vi "Edit Row (Variant).vi"(6 "Row Index":i32, 7 "image path":path, 8 "error in (no error)":errorcluster, 9 "New Row Data (or multi rows)":variant[][](array[variant]), 11 "DataGrid.lvlib:DataTable.lvclass 2":refnum<class "DataTable.lvclass">) -> (0 "error out":errorcluster, 3 "DataGrid.lvlib:DataTable.lvclass 2":refnum<class "DataTable.lvclass">)   [LabVIEW 2013, in "DataGrid.lvlib" / "DataTable.lvclass"]
doc: "Edits a row by simply replacing it with another row (or series of row) to essentially replace and insert at that location in the datatable."
uses:
  DataTable.lvclass
  DataTable.lvclass/DataTable.ctl
  System.Data
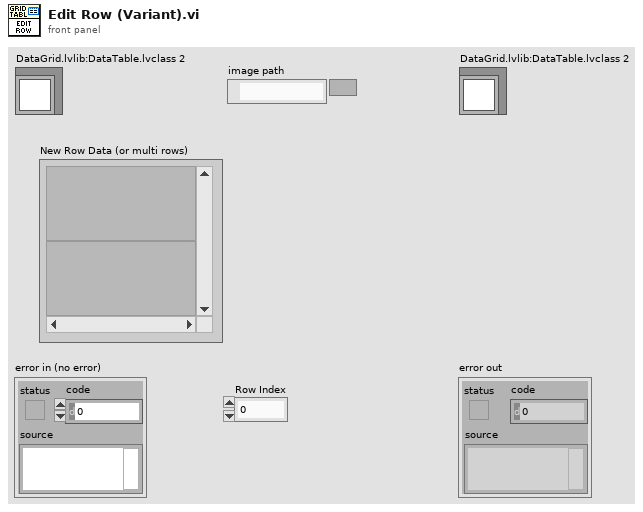
[diagram p1: front panel]
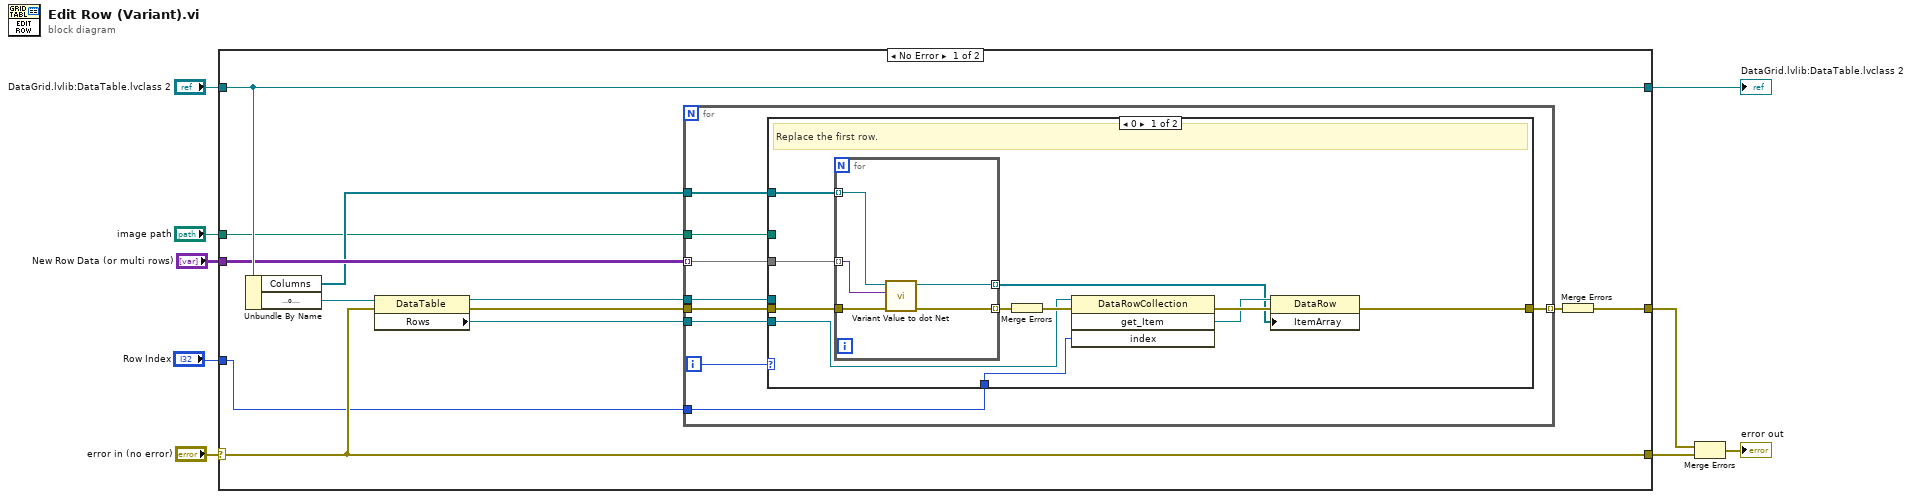
[diagram p0: block diagram]
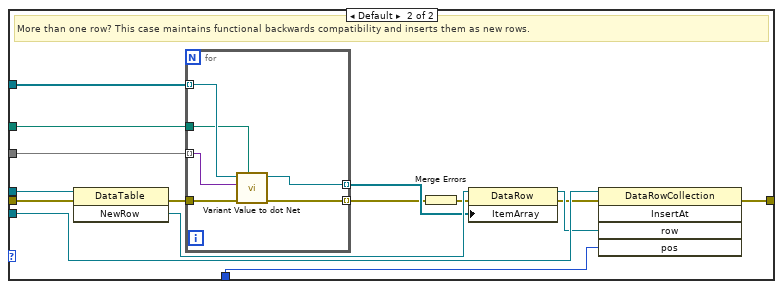
[diagram p2: hidden frame]
diagram:
  n1 = case shown="No Error" "error in (no error)" {
    selector: "error in (no error)" -> [w19 w69]
    tunnel: [w19 w69] -> w8
    tunnel: [w20 w68] -> w6
    tunnel: "DataGrid.lvlib:DataTable.lvclass 2" -> [w20 w68]
    tunnel: "New Row Data (or multi rows)" -> [w18 _]
    tunnel: [w16 _] -> w3
    tunnel: "Row Index" -> [w11 _]
    tunnel: "image path" -> [w10 _]
    frame No Error {
      n2 = Unbundle By Name(w20) -> ("Columns"=w15:refnum<class "GridColumn.lvclass">[], "DataTable"=w17:refnum<k24>)
      n3 = property class="DataTable"(reference=w17, error in=w19) -> (reference out=w14:refnum<k24>, error out=w13:errorcluster, "Rows"=w12:refnum<k24>)
      n4 = for {
        tunnel: w12 -> [w29]
        tunnel: w14 -> [w30]
        tunnel: [w28] -> w21 mode=indexing
        tunnel: w18 -> [w27] mode=indexing
        tunnel: w13 -> [w26]
        tunnel: w15 -> [w25]
        tunnel: w11 -> [w24]
        tunnel: w10 -> [w22]
        i -> [w23]
        n5 = case shown="0" w23 {
          tunnel: w30 -> [_ w61]
          tunnel: w29 -> [w36 w60]
          tunnel: [w31 w59] -> w28
          tunnel: w27 -> [w40 w58]
          tunnel: w26 -> [w39 w50]
          tunnel: w25 -> [w41 w49]
          tunnel: w24 -> [w35 w48]
          tunnel: w22 -> [_ w47]
          frame 0 {
            # "Replace the first row."
            n6 = for {
              tunnel: w40 -> [w46] mode=indexing
              tunnel: [w45] -> w32 mode=indexing
              tunnel: w39 -> [w44]
              tunnel: [w43] -> w38 mode=indexing
              tunnel: w41 -> [w42] mode=indexing
              n7 = call "Variant Value to dot Net.vi"("error in (no error)"=w44, "element"=w46, "GridColumn in"=w42) -> ("error out"=w43:errorcluster, ".NET object"=w45:refnum<k24>)  [unwired: 7 in]
            }
            n8 = Merge Errors(w38) -> (w37:errorcluster)
            n9 = invoke class="DataRowCollection" method="get_Item"(reference=w36, error in=w37, "index"=w35) -> (error out=w34:errorcluster, "get_Item"=w33:refnum<k24>)  [unwired: 1 in, 2 out]
            n10 = property class="DataRow"(reference=w33, error in=w34, "ItemArray"=w32) -> (error out=w31:errorcluster)  [unwired: 1 out]
          }
          frame Default {
            # "More than one row? This case maintains functional backwards compatibility and inserts them as new rows."
            n11 = invoke class="DataTable" method="NewRow"(reference=w61, error in=w50) -> (error out=w57:errorcluster, "NewRow"=w56:refnum<k24>)  [unwired: 1 in, 1 out]
            n12 = for {
              tunnel: w58 -> [w67] mode=indexing
              tunnel: [w66] -> w54 mode=indexing
              tunnel: w57 -> [w65]
              tunnel: [w64] -> w53 mode=indexing
              tunnel: w49 -> [w63] mode=indexing
              tunnel: w47 -> [w62]
              n13 = call "Variant Value to dot Net.vi"("image path"=w62, "error in (no error)"=w65, "element"=w67, "GridColumn in"=w63) -> ("error out"=w64:errorcluster, ".NET object"=w66:refnum<k24>)  [unwired: 6 in]
            }
            n14 = Merge Errors(w53) -> (w52:errorcluster)
            n15 = property class="DataRow"(reference=w56, error in=w52, "ItemArray"=w54) -> (reference out=w55:refnum<k24>, error out=w51:errorcluster)
            n16 = invoke class="DataRowCollection" method="InsertAt"(reference=w60, error in=w51, "row"=w55, "pos"=w48) -> (error out=w59:errorcluster)  [unwired: 1 in, 4 out]
          }
        }
      }
      n17 = Merge Errors(w21) -> (w16:errorcluster)
    }
    frame Error {
    }
  }
  "DataGrid.lvlib:DataTable.lvclass 2" <- w6
  n18 = Merge Errors(w3, w8) -> (→"error out":errorcluster)
